vi "DyMIN_HMI_Main.vi"() -> ()   [LabVIEW 2016]
panel:
  in  "Dwell Time (us)":dbl format="%#_13g"
  out "Initial AOM bits":u16[](array[numeric])
  out "Dwell Time (bits)":u32
  out "Time (bits)":u32[](array[numeric])
  out "Times (us)":dbl[](array[numeric]) min=0.0 max=1.0
  out "AOM bits":u16[](array[numeric])
  out "New File?":bool
  out "File Number":string
  out "Overflow?":bool
  in  "Save Illumination Mask?":bool
  in  "Dymin On?":bool
  in  "Upper Threshold (counts)":u32
  in  "Number of Dymin Steps":u8=1 min=1 max=4 step=1
  in  "AOM Voltage (V)":dbl[](array[numeric])=[0.0, 0.0, 0.0, 0.0] min=0.0 max=1.0
  in  "Times (us)":dbl[](array[numeric])=[0.0, 0.0, 0.0, 0.0] min=0.0 max=10000.0 step=0.0125
  in  "Thresholds (counts)":u32[](array[numeric])
  in  "stop":bool
  # "DyMIN Parameters"
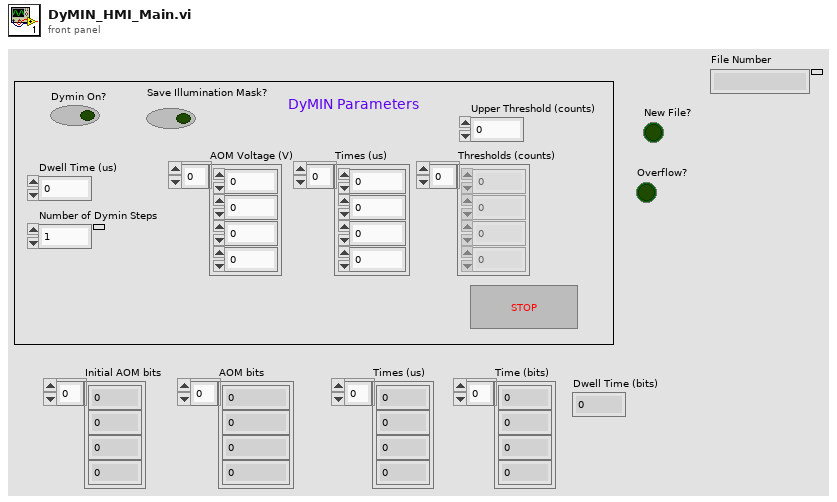
[diagram p1: front panel]
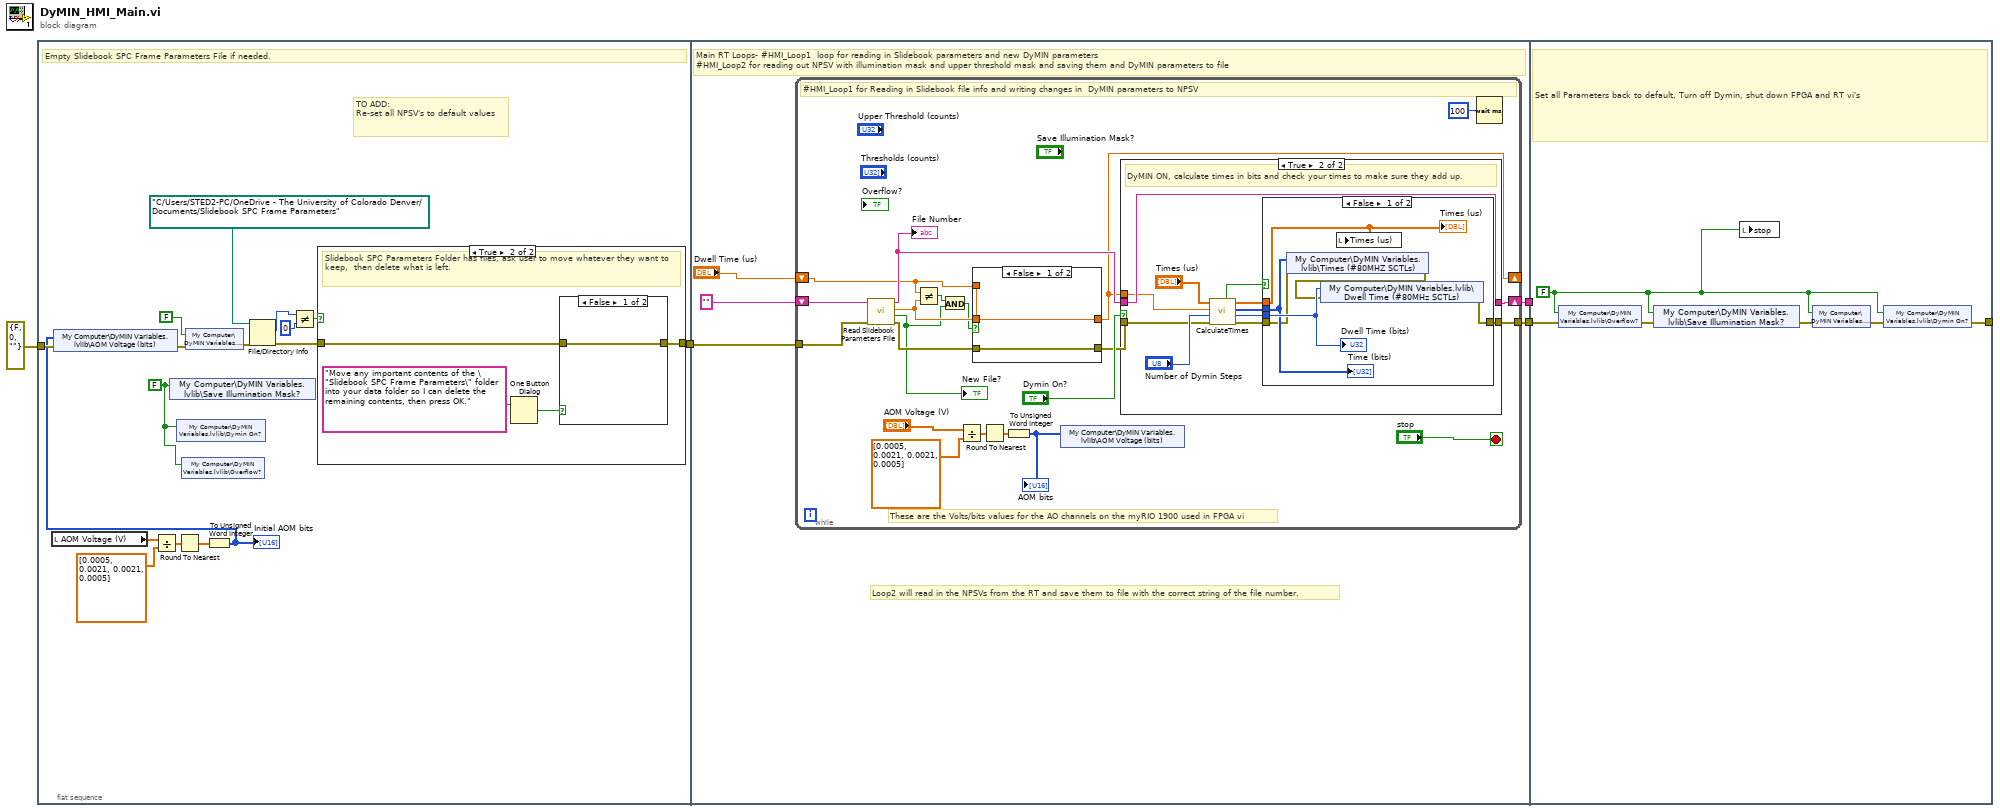
[diagram p0: block diagram]
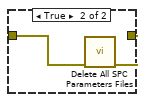
[diagram p3: hidden frame]
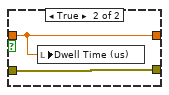
[diagram p4: hidden frame]
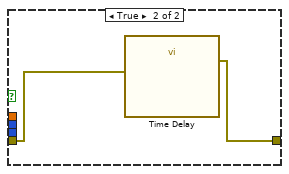
[diagram p6: hidden frame]
diagram:
  n1 = flat-sequence {
    tunnel: errorcluster {"status"=FALSE, "code"=0, "source"=""} ("error in") -> [w9]
    tunnel: [w15] -> w3
    tunnel: w3 -> [w33]
    tunnel: [w32] -> w2
    tunnel: [w30] -> w1
    tunnel: w2 -> [_]
    tunnel: w1 -> [w85]
    tunnel: [w81] -> _
    frame #0 {
      w5 = FALSE ("Save Illumination Mask?")
      # "TO ADD: \nRe-set all NPSV's to default values"
      # "Empty Slidebook SPC Frame Parameters File if needed."
      n2 = local read "AOM Voltage (V)"() -> (w11:dbl[])
      n3 = Divide(x=w11, y=dbl[] [0.0005, 0.0021, 0.0021, 0.0005]) -> (x/y=w14:dbl[])
      n4 = shared-variable "My Computer\\DyMIN Variables.lvlib\\Save Illumination Mask?"(w5) -> ()  [unwired: 1 in, 1 out]
      n5 = shared-variable "My Computer\\DyMIN Variables.lvlib\\Dymin On?"(w5) -> ()  [unwired: 1 in, 1 out]
      n6 = Round To Nearest(number=w14) -> (nearest integer value=w13:dbl[])
      n7 = shared-variable "My Computer\\DyMIN Variables.lvlib\\Overflow?"(w5) -> ()  [unwired: 1 in, 1 out]
      n8 = To Unsigned Word Integer(number=w13) -> (unsigned 16bit integer=w6:u16[])
      "Initial AOM bits" <- w6
      n9 = shared-variable "My Computer\\DyMIN Variables.lvlib\\AOM Voltage (bits)"(w6, error in=w9) -> (error out=w7:errorcluster)
      n10 = shared-variable "My Computer\\DyMIN Variables.lvlib\\Stop"(FALSE ("Stop"), error in=w7) -> (error out=w8:errorcluster)
      n11 = File/Directory Info(path=path "C:/Users/STED2-PC/OneDrive - The University of Colorado Denver/Documents/Slidebook SPC Frame Parameters" ("Folder Path"), error in=w8) -> (size=w19:i64, error out=w16:errorcluster)  [unwired: 5 out]
      n12 = Not Equal?(x=w19, y=i64 0) -> (x != y?=w17:bool)
      n13 = case shown="True" w17 {
        tunnel: w16 -> [w21 w23]
        tunnel: [w21 w22] -> w15
        frame False {
          # "Slidebook SPC Frame Parameters Folder is empty, do nothing"
        }
        frame True {
          # "Slidebook SPC Parameters Folder has files, ask user to move whatever they want to keep,  then delete what is left."
          n14 = One Button Dialog(message="Move any important contents of the \"Slidebook SPC Frame Parameters\" folder into your data folder so I can delete the remaining contents, then press OK.") -> (true=w24:bool)  [unwired: 1 in]
          n15 = case shown="False" w24 {
            tunnel: w23 -> [w26 w28]
            tunnel: [w26 w27] -> w22
            frame False {
            }
            frame True {
              n16 = call "Delete All SPC Parameters Files.vi"("error in (no error)"=w28) -> ("error out"=w27:errorcluster)  [unwired: 10 in]
            }
          }
        }
      }
    }
    frame #1 {
      # "Loop2 will read in the NPSVs from the RT and save them to file with the correct string of the file number."
      # "Main RT Loops- #HMI_Loop1  loop for reading in Slidebook parameters and new DyMIN parameters\n#HMI_Loop2 for reading out NPSV with illumination mask and upper threshold mask and saving them and DyMIN parameters to file"
      n17 = while {
        tunnel: w33 -> [w51]
        shift-right: [w50] -> w32
        shift-left: "" ("File Number Out") -> [w49]
        tunnel: [w48] -> w30
        shift-right: [w39] -> _
        shift-left: "Dwell Time (us)" -> [w38]
        stop <- "stop" stop-if-true
        # "These are the Volts/bits values for the AO channels on the myRIO 1900 used in FPGA vi"
        # "#HMI_Loop1 for Reading in Slidebook file info and writing changes in  DyMIN parameters to NPSV"
        n18 = call "Read Slidebook Parameters File.vi"("error in (no error)"=w51, "File Number In"=w49) -> ("error out"=w41:errorcluster, "New File?"=w35:bool, "Dwell Time (us)"=w37:dbl, "File Number Out"=w52:string)  [unwired: 6 in]
        "File Number" <- w52
        "New File?" <- w35
        n19 = Not Equal?(x=w38, y=w37) -> (x != y?=w36:bool)
        n20 = And(x=w36, y=w35) -> (x .and. y?=w34:bool)
        n21 = Divide(x="AOM Voltage (V)", y=dbl[] [0.0005, 0.0021, 0.0021, 0.0005]) -> (x/y=w43:dbl[])
        n22 = case shown="False" w34 {
          tunnel: [w56 w58] -> w40
          tunnel: w41 -> [w56 w58]
          tunnel: w37 -> [_ w57]
          tunnel: [w55 w57] -> w39
          tunnel: w38 -> [w55 _]
          frame False {
          }
          frame True {
            n23 = local write "Dwell Time (us)"(w57) -> ()
          }
        }
        n24 = Round To Nearest(number=w43) -> (nearest integer value=w44:dbl[])
        n25 = To Unsigned Word Integer(number=w44) -> (unsigned 16bit integer=w47:u16[])
        "AOM bits" <- w47
        n26 = shared-variable "My Computer\\DyMIN Variables.lvlib\\AOM Voltage (bits)"(w47) -> ()  [unwired: 1 in, 1 out]
        n27 = case shown="True" "Dymin On?" {
          tunnel: w52 -> [w60 w66]
          tunnel: [w60 w66] -> w50
          tunnel: w40 -> [w59 w65]
          tunnel: [w59 w62] -> w48
          tunnel: w39 -> [_ w61]
          frame False {
            # "If DyMIN is off, don't do anything"
          }
          frame True {
            # "DyMIN ON, calculate times in bits and check your times to make sure they add up."
            n28 = call "CalculateTimes.vi"("error in"=w65, "Number of Dymin Steps"="Number of Dymin Steps", "Dwell Time (us)"=w61, "Time (us)"="Times (us)") -> ("error out"=w63:errorcluster, "Dwell Time (bits)"=w68:u32, "Time (bits)"=w67:u32[], "Time (us)"=w69:dbl[], "Times F'd up"=w64:bool)  [unwired: 3 in]
            n29 = case shown="False" w64 {
              tunnel: w69 -> [w77 _]
              tunnel: w68 -> [w76 _]
              tunnel: w67 -> [w75 _]
              tunnel: w63 -> [w74 w79]
              tunnel: [w72 w78] -> w62
              frame False {
                n30 = shared-variable "My Computer\\DyMIN Variables.lvlib\\Times (#80MHZ SCTLs)"(w75, error in=w74) -> (error out=w73:errorcluster)
                n31 = shared-variable "My Computer\\DyMIN Variables.lvlib\\Dwell Time (#80MHz SCTLs)"(w76, error in=w73) -> (error out=w72:errorcluster)
                n32 = local write "Times (us)"(w77) -> ()
                "Times (us)" <- w77
                "Time (bits)" <- w75
                "Dwell Time (bits)" <- w76
              }
              frame True {
                n33 = call "Time Delay"("error in (no error)"=w79) -> ("error out"=w78:errorcluster)  [unwired: 10 in]
              }
            }
          }
        }
        n34 = Wait (ms)(milliseconds to wait=u32 100) -> ()  [unwired: 1 out]
      }
    }
    frame #2 {
      w80 = FALSE ("Overflow?")
      # "Set all Parameters back to default, Turn off Dymin, shut down FPGA and RT vi's"
      n35 = shared-variable "My Computer\\DyMIN Variables.lvlib\\Overflow?"(w80, error in=w85) -> (error out=w84:errorcluster)
      n36 = shared-variable "My Computer\\DyMIN Variables.lvlib\\Save Illumination Mask?"(w80, error in=w84) -> (error out=w83:errorcluster)
      n37 = local write "stop"(w80) -> ()
      n38 = shared-variable "My Computer\\DyMIN Variables.lvlib\\Stop"(w80, error in=w83) -> (error out=w82:errorcluster)
      n39 = shared-variable "My Computer\\DyMIN Variables.lvlib\\Dymin On?"(w80, error in=w82) -> (error out=w81:errorcluster)
    }
  }
